vi "LakeShore Read.vi"(1 "Address":string) -> (0 "subarray":dbl[](array[numeric]) format="%.2f")   [LabVIEW 2010]
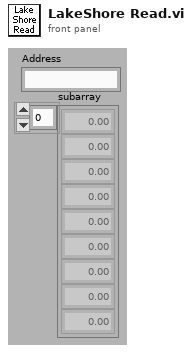
[diagram p1: front panel]
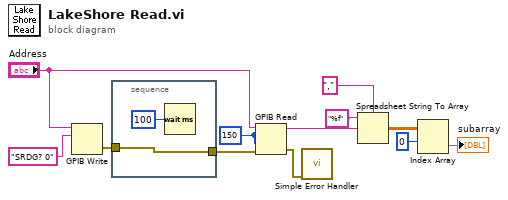
[diagram p0: block diagram]
diagram:
  w12 = 150 ("byte count")
  n1 = GPIB Write(0:"Address", 1:"SRDG? 0") -> (6:w8:errorcluster)  [unwired: 3 in, 1 out]
  n2 = stacked-sequence {
    tunnel: [w14] -> w9
    tunnel: w8 -> [w14]
    frame #0 {
      n3 = Wait (ms)(milliseconds to wait=u32 100) -> ()  [unwired: 1 out]
    }
  }
  n4 = GPIB Read(0:"Address", 1:w12, 2:w12, 3:w9) -> (5:w6:string, 7:w11:errorcluster)  [unwired: 1 in, 1 out]
  n5 = call <vilib>:"Simple Error Handler.vi"("error in (no error)"=w11) -> ()  [unwired: 4 in, 5 out]
  n6 = Spreadsheet String To Array(delimiter (Tab)=",", format string="%f", spreadsheet string=w6) -> (array=w3:dbl[][])  [unwired: 1 in]
  n7 = Index Array(array=w3, index (row)=0) -> (element=→"subarray":dbl[])  [unwired: 1 in]
